vi "VISAInit.vi"(9 "Use DM?":bool, 10 "DM Resource Name":refnum<visa-resource-name> caption="resource name", 11 "Stage Resource Name":refnum<visa-resource-name>) -> (0 "error out":errorcluster, 2 "DM Handle":refnum<visa-resource-name> caption="instrument handle out", 3 "Stage Resource":refnum<visa-resource-name>)   [LabVIEW 2015]
uses:
  <vilib>/Instr/_visa.llb/VISA Configure Serial Port (Instr).vi
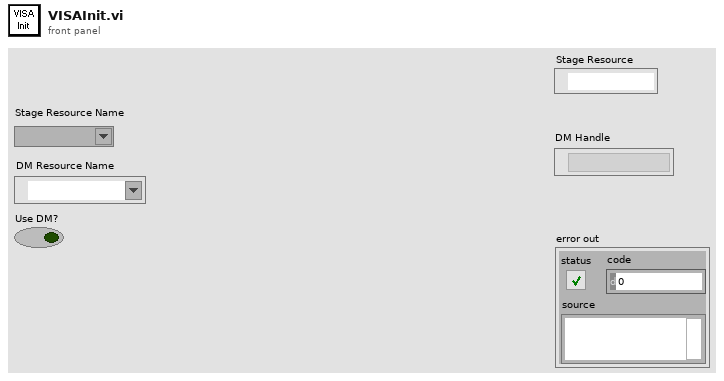
[diagram p1: front panel]
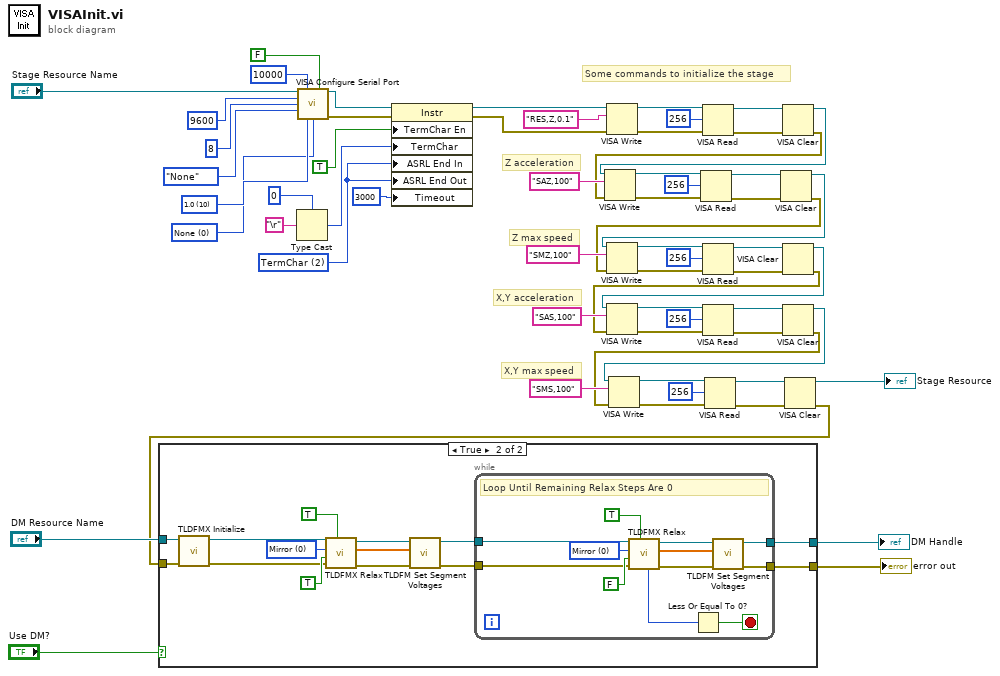
[diagram p0: block diagram]
diagram:
  w48 = u16 2 items=["None", "Last Bit", "TermChar"] ("Serial Settings:End Mode for Reads")
  w56 = u16 0 items=["None", "XON/XOFF", "RTS/CTS", "XON/XOFF & RTS/CTS", "DTR/DSR", "XON/XOFF & DTR/DSR"] ("flow control (0:none)")
  w57 = u16 10 items=["1.0"=10, "1.5"=15, "2.0"=20] ("stop bits (10: 1 bit)")
  # "Z max speed"
  # "X,Y max speed"
  # "X,Y acceleration"
  # "Z acceleration"
  # "Some commands to initialize the stage"
  n1 = Type Cast(type=u8 0 ("Message Based Settings:Termination Character"), x="\r") -> (*(type *) &x=w53:u8)
  n2 = call-poly "VISA Configure Serial Port"("VISA resource name"="Stage Resource Name", "timeout (10sec)"=u32 10000, "Enable Termination\nChar (T)"=FALSE ("Enable Termination\nChar (T)"), "baud rate (9600)"=u32 9600, "data bits (8)"=u16 8, "parity (0:none)"=enum16{"None", "Odd", "Even", "Mark", "Space"}."None", "stop bits (10: 1 bit)"=w57, "flow control (0:none)"=w56) -> ("VISA resource name out"=w52:refnum<visa-resource-name>, "error out"=w51:errorcluster)  [unwired: 6 in]
  n3 = property class="Instr"(reference=w52, error in=w51, "TermChar En"=TRUE ("Message Based Settings:Termination Character Enable"), "TermChar"=w53, "ASRL End In"=w48, "ASRL End Out"=w48, "Timeout"=u32 3000 ("General Settings:Timeout Value")) -> (reference out=w41:refnum<visa-resource-name>, error out=w40:errorcluster)
  n4 = VISA Write(VISA resource name=w41, write buffer="RES,Z,0.1" ("string"), error in (no error)=w40) -> (VISA resource name out=w43:refnum<visa-resource-name>, error out=w44:errorcluster)  [unwired: 1 out]
  n5 = VISA Read(VISA resource name=w43, byte count=u32 256, error in (no error)=w44) -> (VISA resource name out=w46:refnum<visa-resource-name>, error out=w45:errorcluster)  [unwired: 2 out]
  n6 = VISA Clear(VISA resource name=w46, error in (no error)=w45) -> (VISA resource name out=w12:refnum<visa-resource-name>, error out=w14:errorcluster)
  n7 = VISA Write(VISA resource name=w12, write buffer="SAZ,100" ("string"), error in (no error)=w14) -> (VISA resource name out=w35:refnum<visa-resource-name>, error out=w36:errorcluster)  [unwired: 1 out]
  n8 = VISA Read(VISA resource name=w35, byte count=u32 256, error in (no error)=w36) -> (VISA resource name out=w38:refnum<visa-resource-name>, error out=w37:errorcluster)  [unwired: 2 out]
  n9 = VISA Clear(VISA resource name=w38, error in (no error)=w37) -> (VISA resource name out=w11:refnum<visa-resource-name>, error out=w13:errorcluster)
  n10 = VISA Write(VISA resource name=w11, write buffer="SMZ,100" ("string"), error in (no error)=w13) -> (VISA resource name out=w30:refnum<visa-resource-name>, error out=w29:errorcluster)  [unwired: 1 out]
  n11 = VISA Read(VISA resource name=w30, byte count=u32 256, error in (no error)=w29) -> (VISA resource name out=w27:refnum<visa-resource-name>, error out=w28:errorcluster)  [unwired: 2 out]
  n12 = VISA Clear(VISA resource name=w27, error in (no error)=w28) -> (VISA resource name out=w9:refnum<visa-resource-name>, error out=w10:errorcluster)
  n13 = VISA Write(VISA resource name=w9, write buffer="SAS,100" ("string"), error in (no error)=w10) -> (VISA resource name out=w23:refnum<visa-resource-name>, error out=w24:errorcluster)  [unwired: 1 out]
  n14 = VISA Read(VISA resource name=w23, byte count=u32 256, error in (no error)=w24) -> (VISA resource name out=w26:refnum<visa-resource-name>, error out=w25:errorcluster)  [unwired: 2 out]
  n15 = VISA Clear(VISA resource name=w26, error in (no error)=w25) -> (VISA resource name out=w8:refnum<visa-resource-name>, error out=w7:errorcluster)
  n16 = VISA Write(VISA resource name=w8, write buffer="SMS,100" ("string"), error in (no error)=w7) -> (VISA resource name out=w18:refnum<visa-resource-name>, error out=w17:errorcluster)  [unwired: 1 out]
  n17 = VISA Read(VISA resource name=w18, byte count=u32 256, error in (no error)=w17) -> (VISA resource name out=w15:refnum<visa-resource-name>, error out=w16:errorcluster)  [unwired: 2 out]
  n18 = VISA Clear(VISA resource name=w15, error in (no error)=w16) -> (VISA resource name out=→"Stage Resource":refnum<visa-resource-name>, error out=w4:errorcluster)
  n19 = case shown="True" "Use DM?" {
    tunnel: "DM Resource Name" -> [w63 w78]
    tunnel: w4 -> [w64 w77]
    tunnel: [w63 w66] -> w3
    tunnel: [w64 w65] -> w2
    frame False {
    }
    frame True {
      w69 = u32 0 items=["Mirror", "Arms", "Mirror + Arms"] ("Device Part (Mirror)")
      n20 = call "TLDFMX Initialize.vi"("error in (no error)"=w77, "resource name"=w78) -> ("error out"=w67:errorcluster, "instrument handle out"=w68:refnum<visa-resource-name>)  [unwired: 8 in]
      n21 = call "TLDFMX Relax.vi"("Reload (1)"=TRUE, "error in (no error)"=w67, "Is First Step (0)"=TRUE, "Device Part (Mirror)"=w69, "instrument handle"=w68) -> ("error out"=w73:errorcluster, "Relax Pattern Mirror (0)"=w74:dbl[], "instrument handle out"=w72:refnum<visa-resource-name>)  [unwired: 2 in, 2 out]
      n22 = call "TLDFM Set Segment Voltages.vi"("error in (no error)"=w73, "Segment Voltages"=w74, "instrument handle"=w72) -> ("error out"=w76:errorcluster, "instrument handle out"=w75:refnum<visa-resource-name>)  [unwired: 7 in]
      n23 = while {
        tunnel: w75 -> [w84]
        tunnel: w76 -> [w83]
        tunnel: [w80] -> w66
        tunnel: [w79] -> w65
        stop <- w81 stop-if-true
        w85 = u32 0 items=["Mirror", "Arms", "Mirror + Arms"] ("Device Part (Mirror)")
        # "Loop Until Remaining Relax Steps Are 0"
        n24 = call "TLDFMX Relax.vi"("Reload (1)"=TRUE, "error in (no error)"=w83, "Is First Step (0)"=FALSE, "Device Part (Mirror)"=w85, "instrument handle"=w84) -> ("error out"=w89:errorcluster, "Relax Pattern Mirror (0)"=w90:dbl[], "instrument handle out"=w88:refnum<visa-resource-name>, "Remaining Steps"=w82:i32)  [unwired: 2 in, 1 out]
        n25 = Less Or Equal To 0?(x=w82) -> (x <= 0?=w81:bool)
        n26 = call "TLDFM Set Segment Voltages.vi"("error in (no error)"=w89, "Segment Voltages"=w90, "instrument handle"=w88) -> ("error out"=w79:errorcluster, "instrument handle out"=w80:refnum<visa-resource-name>)  [unwired: 7 in]
      }
    }
  }
  "error out" <- w2
  "DM Handle" <- w3
